vi "3D Scanner - Servo - AUTO.vi"() -> ()   [LabVIEW 2012]
uses:
  <vilib>/Instr/_visa.llb/VISA Configure Serial Port (Instr).vi
panel:
  in  "Select COM Port Pololu":refnum<visa-resource-name>="COM4"
  # "3D Scanner servo Controller"
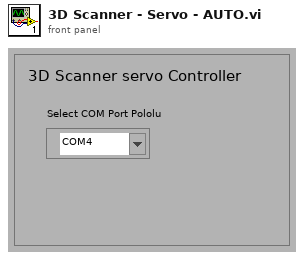
[diagram p1: front panel]
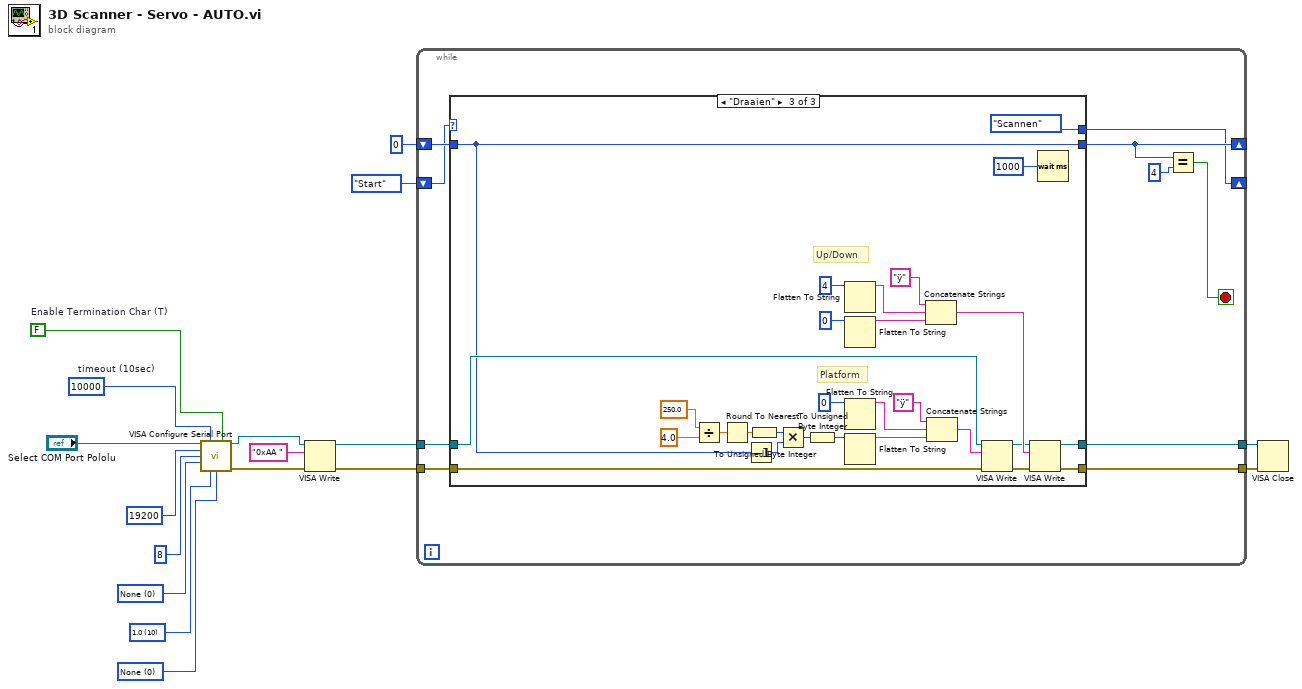
[diagram p0: block diagram]
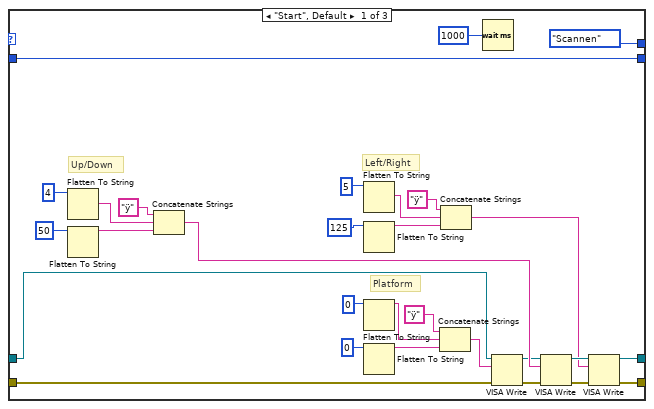
[diagram p2: hidden frame]
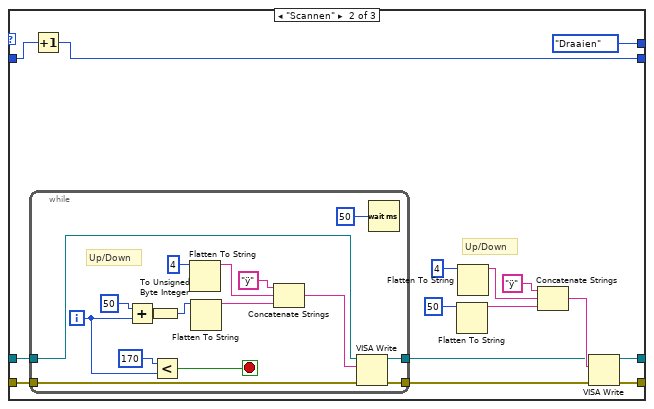
[diagram p3: hidden frame]
diagram:
  w13 = u16 0 items=["None"=0, "XON/XOFF"=1, "RTS/CTS"=2, "DTR/DSR"=4] ("flow control")
  w12 = u16 10 items=["1.0"=10, "1.5"=15, "2.0"=20] ("stop bits")
  w11 = u16 0 items=["None", "Odd", "Even", "Mark", "Space"] ("parity")
  w8 = FALSE  # Enable Termination Char (T)
  w7 = u32 10000  # timeout (10sec)
  n1 = call-poly "VISA Configure Serial Port"("VISA resource name"="Select COM Port Pololu", "timeout (10sec)"=w7, "Enable Termination\nChar (T)"=w8, "baud rate (9600)"=u32 19200 ("baud rate"), "data bits (8)"=u16 8 ("data bits"), "parity (0:none)"=w11, "stop bits (10: 1 bit)"=w12, "flow control (0:none)"=w13) -> ("VISA resource name out"=w15:refnum<visa-resource-name>, "error out"=w14:errorcluster)  [unwired: 1 in, 5 out]
  n2 = VISA Write(VISA resource name=w15, write buffer="0xAA ", error in (no error)=w14) -> (VISA resource name out=w5:refnum<visa-resource-name>, error out=w4:errorcluster)  [unwired: 1 out]
  n3 = while {
    tunnel: w4 -> [w27]
    tunnel: w5 -> [w26]
    tunnel: [w25] -> w17
    tunnel: [w24] -> w16
    shift-right: [w21] -> _
    shift-left: u8 0 -> [w23]
    shift-right: [w19] -> _
    shift-left: enum16{"Start", "Scannen", "Draaien"}."Start" -> [w18]
    stop <- w22 stop-if-true
    n4 = case shown="\"Draaien\"" w18 {
      tunnel: w27 -> [w36 w62 w103]
      tunnel: w26 -> [w35 w63 w102]
      tunnel: [w32 w65 w94] -> w25
      tunnel: [w31 w64 w93] -> w24
      tunnel: w23 -> [w30 w59 w89]
      tunnel: [w30 w58 w89] -> w21
      tunnel: [enum16{"Start", "Scannen", "Draaien"}."Scannen" enum16{"Start", "Scannen", "Draaien"}."Draaien" enum16{"Start", "Scannen", "Draaien"}."Scannen"] -> w19
      frame "Start", Default {
        # "Left/Right"
        # "Up/Down"
        # "Platform"
        n5 = Flatten To String(anything=u8 4) -> (data string=w51:string)  [unwired: 1 in, 4 out]
        n6 = Flatten To String(anything=u8 50) -> (data string=w50:string)  [unwired: 1 in, 4 out]
        n7 = Concatenate Strings("ÿ", w51, w50) -> (w43:string)
        n8 = Flatten To String(anything=u8 5) -> (data string=w55:string)  [unwired: 1 in, 4 out]
        n9 = Flatten To String(anything=u8 125) -> (data string=w54:string)  [unwired: 1 in, 4 out]
        n10 = Flatten To String(anything=u8 0) -> (data string=w47:string)  [unwired: 1 in, 4 out]
        n11 = Flatten To String(anything=u8 0) -> (data string=w46:string)  [unwired: 1 in, 4 out]
        n12 = Concatenate Strings("ÿ", w47, w46) -> (w44:string)
        n13 = Concatenate Strings("ÿ", w55, w54) -> (w40:string)
        n14 = Wait (ms)(milliseconds to wait=u32 1000) -> ()  [unwired: 1 out]
        n15 = VISA Write(VISA resource name=w35, write buffer=w44, error in (no error)=w36) -> (VISA resource name out=w42:refnum<visa-resource-name>, error out=w34:errorcluster)  [unwired: 1 out]
        n16 = VISA Write(VISA resource name=w42, write buffer=w43, error in (no error)=w34) -> (VISA resource name out=w41:refnum<visa-resource-name>, error out=w33:errorcluster)  [unwired: 1 out]
        n17 = VISA Write(VISA resource name=w41, write buffer=w40, error in (no error)=w33) -> (VISA resource name out=w32:refnum<visa-resource-name>, error out=w31:errorcluster)  [unwired: 1 out]
      }
      frame "Scannen" {
        # "Up/Down"
        n18 = while {
          tunnel: w63 -> [w80]
          tunnel: w62 -> [w79]
          tunnel: [w78] -> w61
          tunnel: [w77] -> w60
          i -> [w73]
          stop <- w87 stop-if-true
          # "Up/Down"
          n19 = Add(x=50, y=w73) -> (x+y=w74:i32)
          n20 = To Unsigned Byte Integer(number=w74) -> (unsigned 8bit integer=w76:u8)
          n21 = Less?(x=170, y=w73) -> (x < y?=w87:bool)
          n22 = Flatten To String(anything=u8 4) -> (data string=w83:string)  [unwired: 1 in, 4 out]
          n23 = Flatten To String(anything=w76) -> (data string=w84:string)  [unwired: 2 in, 3 out]
          n24 = Concatenate Strings("ÿ", w83, w84) -> (w81:string)
          n25 = VISA Write(VISA resource name=w80, write buffer=w81, error in (no error)=w79) -> (VISA resource name out=w78:refnum<visa-resource-name>, error out=w77:errorcluster)  [unwired: 1 out]
          n26 = Wait (ms)(milliseconds to wait=u32 50) -> ()  [unwired: 1 out]
        }
        n27 = Increment(x=w59) -> (x+1=w58:u8)
        n28 = Flatten To String(anything=u8 50) -> (data string=w69:string)  [unwired: 1 in, 4 out]
        n29 = Flatten To String(anything=u8 4) -> (data string=w70:string)  [unwired: 1 in, 4 out]
        n30 = Concatenate Strings("ÿ", w70, w69) -> (w67:string)
        n31 = VISA Write(VISA resource name=w61, write buffer=w67, error in (no error)=w60) -> (VISA resource name out=w65:refnum<visa-resource-name>, error out=w64:errorcluster)  [unwired: 1 out]
      }
      frame "Draaien" {
        # "Up/Down"
        # "Platform"
        n32 = Divide(x=250.0, y=4.0) -> (x/y=w97:dbl)
        n33 = Round To Nearest(number=w97) -> (nearest integer value=w98:dbl)
        n34 = Decrement(x=w89) -> (x-1=w88:u8)
        n35 = To Unsigned Byte Integer(number=w98) -> (unsigned 8bit integer=w99:u8)
        n36 = Multiply(x=w99, y=w88) -> (x*y=w92:u8)
        n37 = To Unsigned Byte Integer(number=w92) -> (unsigned 8bit integer=w91:u8)
        n38 = Flatten To String(anything=u8 4) -> (data string=w114:string)  [unwired: 1 in, 4 out]
        n39 = Flatten To String(anything=u8 0) -> (data string=w113:string)  [unwired: 1 in, 4 out]
        n40 = Flatten To String(anything=u8 0) -> (data string=w110:string)  [unwired: 1 in, 4 out]
        n41 = Flatten To String(anything=w91) -> (data string=w109:string)  [unwired: 1 in, 4 out]
        n42 = Concatenate Strings("ÿ", w114, w113) -> (w106:string)
        n43 = Concatenate Strings("ÿ", w110, w109) -> (w107:string)
        n44 = VISA Write(VISA resource name=w102, write buffer=w107, error in (no error)=w103) -> (VISA resource name out=w105:refnum<visa-resource-name>, error out=w101:errorcluster)  [unwired: 1 out]
        n45 = VISA Write(VISA resource name=w105, write buffer=w106, error in (no error)=w101) -> (VISA resource name out=w94:refnum<visa-resource-name>, error out=w93:errorcluster)  [unwired: 1 out]
        n46 = Wait (ms)(milliseconds to wait=u32 1000) -> ()  [unwired: 1 out]
      }
    }
    n47 = Equal?(x=w21, y=u8 4) -> (x = y?=w22:bool)
  }
  n48 = VISA Close(VISA resource name=w17, error in (no error)=w16) -> ()  [unwired: 1 out]
